vi "dfd_Dummy_INT Gain Processing.vi"(1 "x":i32) -> (0 "y":i32)   [LabVIEW 2017]
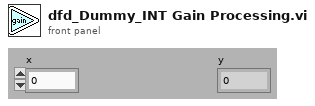
[diagram p1: front panel]
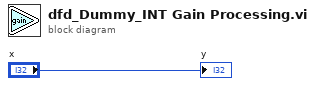
[diagram p0: block diagram]
diagram:
  "y" <- "x"
